vi "RoadkillMain.vi"() -> ()   [LabVIEW 2014]
uses:
  Command.ctl
  DataHighway.ctl
  <vilib>/myRIO/Common/Instrument Driver Framework/myRIO v1.0/UART/vis/myRIO v1.0 Close UART.vi
  <vilib>/myRIO/Common/Instrument Driver Framework/Utilities/vis/FPGA Ref Manager.vi
  <vilib>/myRIO/Common/Instrument Driver Framework/myRIO v1.0/myRIO v1.0 Reset FPGA.vi
  <vilib>/myRIO/Common/Instrument Driver Framework/myRIO v1.0/IRQ/vis/myRIO v1.0 IRQ Info FGV.vi
  <vilib>/myRIO/Common/Instrument Driver Framework/myRIO v1.0/IRQ/vis/myRIO v1.0 Timer IRQ Info FGV.vi
  <vilib>/myRIO/Common/Instrument Driver Framework/myRIO v1.0/IRQ/vis/myRIO v1.0 ISR Agent.vi
  <vilib>/ErrorRing/Error Ring.xnode
  <vilib>/myRIO/Instrument Drivers/Utilities/Utilities.lvlib
panel:
  out "Step Position":dbl
  out "DataHWay":T1
  out "ComHWayFromOCU":T2 {"Speed" scale=-2.0..10.0; "Rudder" scale=-10.0..10.0}
  in  "stop robot control":bool
  out "error out":errorcluster
  # "Robot will run headless\nwithout a control panel\nso keep this control panel\nas simple as possible while\nstill allowing debugging."
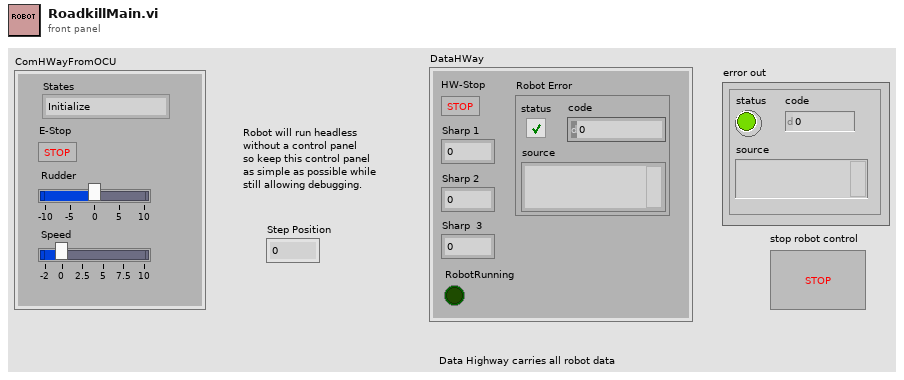
[diagram p1: front panel]
types:
  T1 = typedef "DataHighway.ctl" = cluster{"HW-Stop":bool, "Sharp 1":dbl, "Sharp 2":dbl, "Sharp  3":dbl, "RobotRunning":bool, "Robot Error":errorcluster}
  T2 = typedef "Command.ctl" = cluster{"States":enum16{"Initialize", "Wait for Event", "Debug Robot", "Run Robot", "Exit"}, "E-Stop":bool, "Rudder":dbl, "Speed":dbl}
  T3 = enum16{"Initialize", "Wait for Event", "Debug Robot", "Run Robot", "Exit"}
  T4 = cluster{"LED0":bool, "LED0 1":bool, "LED0 2":bool}
  T5 = cluster{"Port":dbl, "Center":dbl, "Starboard":dbl}
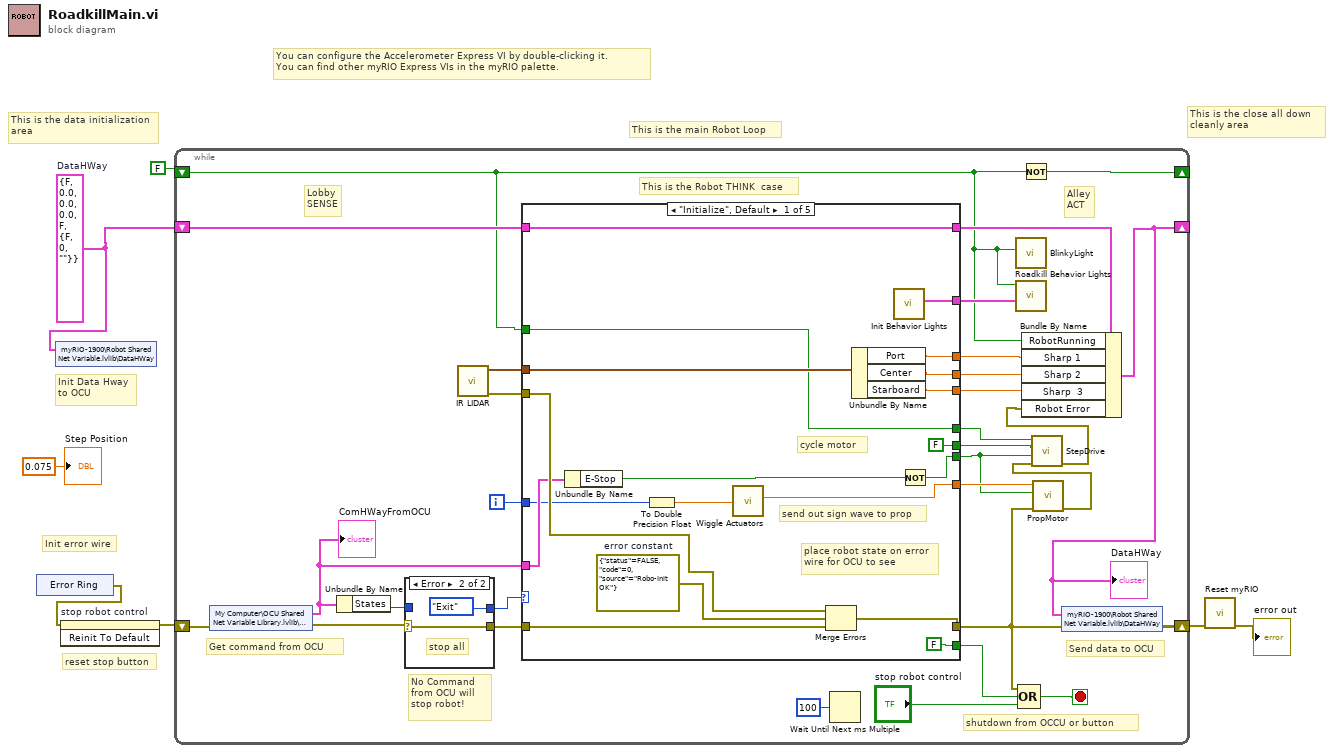
[diagram p0: block diagram]
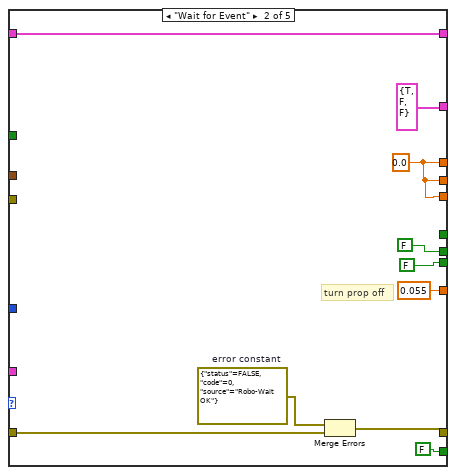
[diagram p3: hidden frame]
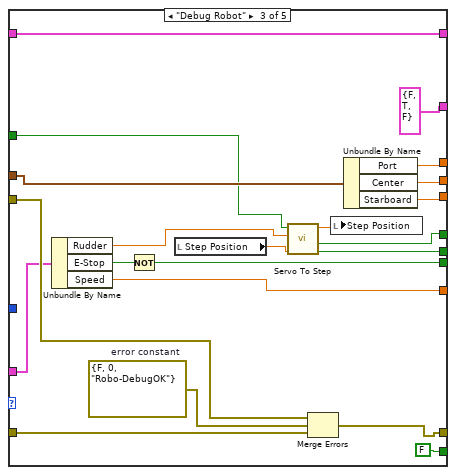
[diagram p4: hidden frame]
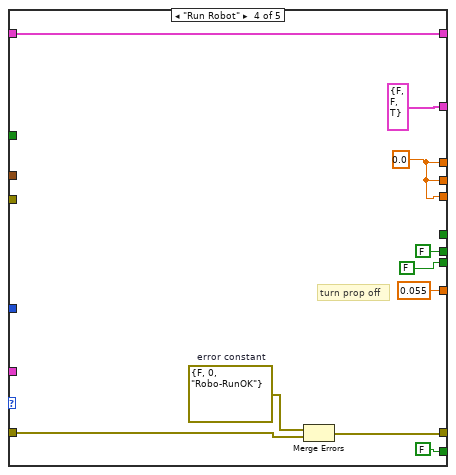
[diagram p5: hidden frame]
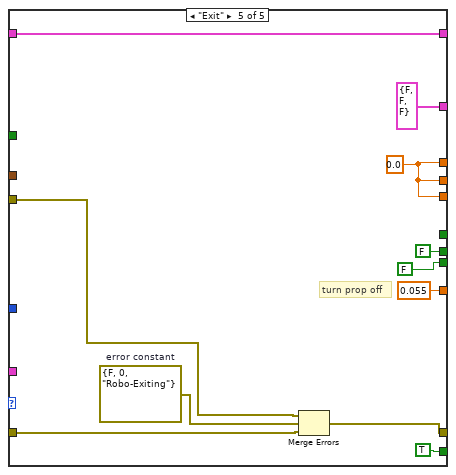
[diagram p6: hidden frame]
diagram:
  w4 = T1 {"HW-Stop"=FALSE, "Sharp 1"=0.0, "Sharp 2"=0.0, "Sharp  3"=0.0, "RobotRunning"=FALSE, "Robot Error"={"status"=FALSE, "code"=0, "source"=""}}  # DataHWay
  # "reset stop button"
  # "Init error wire"
  # "Init Data Hway\nto OCU"
  # "This is the close all down \ncleanly area"
  # "This is the data initialization\narea"
  # "This is the main Robot Loop"
  # "You can configure the Accelerometer Express VI by double-clicking it.\nYou can find other myRIO Express VIs in the myRIO palette."
  n1 = xnode "Error Ring"() -> ("error out"=w3:errorcluster)
  n2 = shared-variable "myRIO-1900\\Robot Shared Net Variable.lvlib\\DataHWay"(w4) -> ()  [unwired: 1 in, 1 out]
  n3 = invoke on="stop robot control" class="Bool" method="Reinit To Default"(error in=w3) -> (error out=w2:errorcluster)  [unwired: 2 in, 2 out]
  n4 = while {
    shift-right: [w28] -> w6
    shift-left: w2 -> [w25]
    shift-right: [w23] -> _
    shift-left: w4 -> [w32]
    shift-right: [w27] -> _
    shift-left: FALSE -> [w13]
    i -> [w9]
    stop <- w35 stop-if-true
    # "No Command \nfrom OCU will\nstop robot!"
    # "Get command from OCU"
    # "Send data to OCU"
    # "shutdown from OCCU or button"
    # "Alley\nACT"
    # "This is the Robot THINK  case"
    # "Lobby\nSENSE"
    n5 = shared-variable "My Computer\\OCU Shared Net Variable Library.lvlib\\ComHWay"(error in=w25) -> (w29:T2, error out=w24:errorcluster)
    "ComHWayFromOCU" <- w29
    n6 = Unbundle By Name(w29) -> ("States"=w30:T3)
    n7 = case shown="Error" w24 {
      selector: w24 -> [w39 w41]
      tunnel: [w39 w41] -> w36
      tunnel: [w38 T3."Exit" ("States")] -> w37
      tunnel: w30 -> [w38 _]
      frame No Error {
      }
      frame Error {
        # "stop all"
      }
    }
    n8 = call "IR LIDAR.vi"() -> ("error out"=w20:errorcluster, "Range"=w21:T5)  [unwired: 10 in]
    n9 = case shown="\"Initialize\", Default" w37 {
      tunnel: w36 -> [w58 w68 w89 w99 w110]
      tunnel: [w57 w67 w88 w98 w109] -> w12
      tunnel: [FALSE FALSE FALSE FALSE TRUE] -> w34
      tunnel: w32 -> [w59 w69 w91 w101 w111]
      tunnel: [w59 w69 w91 w101 w111] -> w26
      tunnel: w29 -> [w49 _ w80 _ _]
      tunnel: [w55 T4 {"LED0"=TRUE, "LED0 1"=FALSE, "LED0 2"=FALSE} ("Behavior Lights In") T4 {"LED0"=FALSE, "LED0 1"=TRUE, "LED0 2"=FALSE} ("Behavior Lights In") T4 {"LED0"=FALSE, "LED0 1"=FALSE, "LED0 2"=TRUE} ("Behavior Lights In") T4 {"LED0"=FALSE, "LED0 1"=FALSE, "LED0 2"=FALSE} ("Behavior Lights In")] -> w22
      tunnel: w21 -> [w53 _ w84 _ _]
      tunnel: w20 -> [w54 _ w85 _ w105]
      tunnel: [w52 w64 w83 w95 w106] -> w19
      tunnel: [w51 w64 w82 w95 w106] -> w18
      tunnel: [w50 w64 w81 w95 w106] -> w17
      tunnel: [w48 FALSE ("E-Stop") w75 FALSE ("E-Stop") FALSE ("E-Stop")] -> w8
      tunnel: [FALSE ("Direction") FALSE ("Direction") w77 FALSE ("Direction") FALSE ("Direction")] -> w15
      tunnel: [w43 _ w74 _ _] -> w14
      tunnel: w13 -> [w43 _ w73 _ _]
      tunnel: [w46 0.055 ("Speed") w71 0.055 ("Speed") 0.055 ("Speed")] -> w10
      tunnel: w9 -> [w45 _ _ _ _]
      frame "Initialize", Default {
        w56 = errorcluster {"status"=FALSE, "code"=0, "source"="Robo-Init OK"}  # error constant
        # "cycle motor"
        # "send out sign wave to prop"
        # "place robot state on error\nwire for OCU to see"
        n10 = Unbundle By Name "Unbundle By Name"(w49) -> ("E-Stop"=w47:bool)
        n11 = To Double Precision Float(number=w45) -> (double precision float=w44:dbl)
        n12 = call "Wiggle Actuators.vi"("Trigger"=w44) -> ("MotorCommand"=w46:dbl)  [unwired: 10 in]
        n13 = Merge Errors "Merge Errors"(w54, w56, w58) -> (w57:errorcluster)
        n14 = Unbundle By Name(w53) -> ("Port"=w52:dbl, "Center"=w51:dbl, "Starboard"=w50:dbl)
        n15 = call "Init Behavior Lights.vi"() -> ("Lights Out"=w55:cluster{"Red":bool, "Blue":bool, "Green":bool})  [unwired: 11 in]
        n16 = Not(x=w47) -> (.not. x?=w48:bool)
      }
      frame "Wait for Event" {
        w64 = 0.0 ("Port")
        w66 = errorcluster {"status"=FALSE, "code"=0, "source"="Robo-Wait OK"}  # error constant
        # "turn prop off"
        n17 = Merge Errors "Merge Errors"(w66, w68) -> (w67:errorcluster)
      }
      frame "Debug Robot" {
        w87 = errorcluster {"status"=FALSE, "code"=0, "source"="Robo-DebugOK"}  # error constant
        n18 = Unbundle By Name "Unbundle By Name"(w80) -> ("Rudder"=w72:dbl, "E-Stop"=w79:bool, "Speed"=w71:dbl)
        n19 = Not(x=w79) -> (.not. x?=w75:bool)
        n20 = local read "Step Position"() -> (w78:dbl)
        n21 = call "Servo To Step.vi"("Step Position"=w78, "Rudder"=w72, "Step"=w73) -> ("Direction"=w77:bool, "Step"=w74:bool, "New Position"=w76:dbl)  [unwired: 6 in]
        n22 = Merge Errors "Merge Errors"(w85, w87, w89) -> (w88:errorcluster)
        n23 = local write "Step Position"(w76) -> ()
        n24 = Unbundle By Name(w84) -> ("Port"=w83:dbl, "Center"=w82:dbl, "Starboard"=w81:dbl)
      }
      frame "Run Robot" {
        w95 = 0.0 ("Port")
        w97 = errorcluster {"status"=FALSE, "code"=0, "source"="Robo-RunOK"}  # error constant
        # "turn prop off"
        n25 = Merge Errors "Merge Errors"(w97, w99) -> (w98:errorcluster)
      }
      frame "Exit" {
        w106 = 0.0 ("Port")
        w108 = errorcluster {"status"=FALSE, "code"=0, "source"="Robo-Exiting"}  # error constant
        # "turn prop off"
        n26 = Merge Errors "Merge Errors"(w105, w108, w110) -> (w109:errorcluster)
      }
    }
    n27 = Wait Until Next ms Multiple(millisecond multiple=u32 100) -> ()  [unwired: 1 out]
    n28 = call "BlinkyLight.vi"("Light In"=w13) -> ()  [unwired: 11 in]
    n29 = call "Roadkill Behavior Lights.vi"("Behavior Lights In"=w22, "Blink"=w13) -> ()  [unwired: 10 in]
    n30 = Compound Arithmetic op=OR(w12, w34, "stop robot control") -> (w35:bool)
    n31 = Not(x=w13) -> (.not. x?=w27:bool)
    n32 = call "PropMotor.vi"("error in (no error)"=w12, "E-Stop"=w8, "Prop Speed"=w10) -> ("error out"=w11:errorcluster)  [unwired: 8 in]
    n33 = call "StepDrive.vi"("error in (no error)"=w11, "Enable"=w8, "Direction"=w15, "Step"=w14) -> ("error out"=w16:errorcluster)  [unwired: 7 in]
    n34 = Bundle By Name(cluster=w26, "RobotRunning"=w13, "Sharp 1"=w19, "Sharp 2"=w18, "Sharp  3"=w17, "Robot Error"=w16) -> (w23:T1)
    "DataHWay" <- w23
    n35 = shared-variable "myRIO-1900\\Robot Shared Net Variable.lvlib\\DataHWay"(w23, error in=w12) -> (error out=w28:errorcluster)
  }
  n36 = call <vilib>:"Reset myRIO.vi"("error in (no error)"=w6) -> ("error out"=→"error out":errorcluster)  [unwired: 10 in]
  "Step Position" <- 0.075 ("Step Position")
